vi "Get Over Voltage Protection State.vi"(8 "error in (no error)":errorcluster, 11 "VISA resource name":refnum<visa-resource-name>) -> (0 "error out":errorcluster, 1 "Source Voltage Protection State?":bool, 3 "VISA resource name out":refnum<visa-resource-name>)   [LabVIEW 2022 SP3, in "Keithley 2450.lvlib"]
doc: "This command indicates if the overvoltage source protection feature is active"
uses:
  Keithley 2450.lvlib
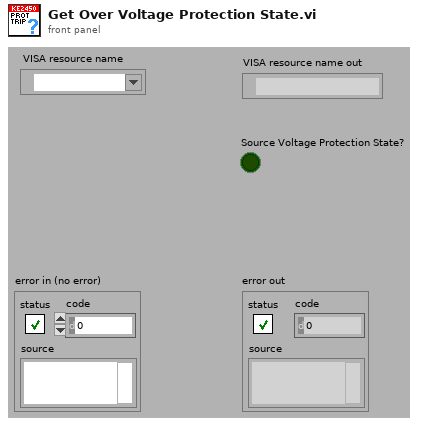
[diagram p1: front panel]
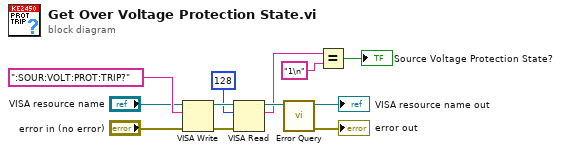
[diagram p0: block diagram]
diagram:
  n1 = VISA Write(VISA resource name="VISA resource name", write buffer=":SOUR:VOLT:PROT:TRIP?", error in (no error)="error in (no error)") -> (VISA resource name out=w9:refnum<visa-resource-name>, error out=w10:errorcluster)  [unwired: 1 out]
  n2 = VISA Read(VISA resource name=w9, byte count=u32 128, error in (no error)=w10) -> (VISA resource name out=w7:refnum<visa-resource-name>, read buffer=w3:string)  [unwired: 2 out]
  n3 = call "Error Query.vi"("VISA resource name"=w7) -> ("error out"=→"error out":errorcluster, "VISA resource name out"=→"VISA resource name out":refnum<visa-resource-name>)  [unwired: 1 in, 8 out]
  n4 = Equal?(x=w3, y="1\n") -> (x = y?=→"Source Voltage Protection State?":bool)
